vi "Inline - Update Status Channels.vi"(7 "Status Channel":T1, 8 "Error Code":i32, 9 "Time (us)":u32, 11 "RTStateVariables":T2 {"Inline Status Channels Refs" format="%.0x"; "Rx Config"."Labels Settings"."Label Timestamp Channel Data Reference" format="%.0x"; "Rx Config"."Labels Settings"."Label Disable/Trigger Channel Reference" format="%.0x"; "Rx Config"."Labels Settings"."Label" format="%.0o"}) -> ()   [LabVIEW 2020, in "Ballard Arinc-429 Engine.lvlib"]
doc: "This VI updates some Inline Status Channels."
uses:
  Ballard Arinc-429 Engine.lvlib
  RT Controls/RTStateVariables.ctl
  <vilib>/NI/NIVS Inline Async API/_VS Inline Async API/VS Inline Async API/VS Inline Async API.lvclass
  RT Controls/Card Parameters.ctl
  Shared/Controls and Global/Initialization Method.ctl
  Shared/Controls and Global/RT HW Channel.ctl
  Shared/Controls and Global/RT Label Settings.ctl
  Shared/Controls and Global/Label.ctl
  Shared/Controls and Global/transferPeriod.ctl
  Shared/Controls and Global/RT Word Settings.ctl
  Shared/Controls and Global/RT Param Setting.ctl
  Shared/Controls and Global/Start Bit.ctl
  Shared/Controls and Global/Number of Bits.ctl
  <vilib>/NI VeriStand/Custom Device API/Block Data Reference.ctl
  <vilib>/NI VeriStand/Custom Device API/Data Reference.ctl
  <vilib>/NI VeriStand/Custom Device API/Custom Device Item Ref.ctl
  Shared/Controls and Global/TransferType.ctl
  RT Controls/Inline_Status_Channels.ctl
  <vilib>/NI VeriStand/Custom Device API/Global Data Refs.vi
  <vilib>/NI VeriStand/Custom Device API/Custom Device API.lvlib
  Shared/Ballard Arinc-429 Shared.lvlib
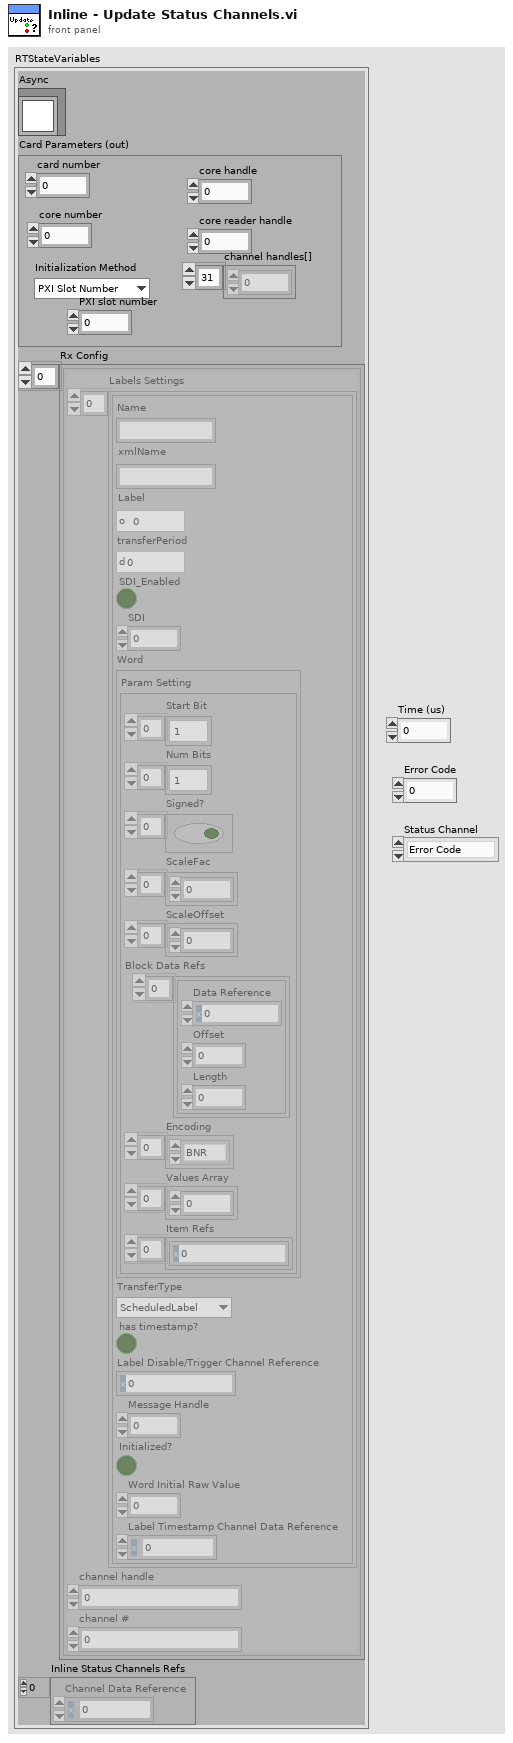
[diagram p1: front panel]
types:
  T1 = typedef "Ballard Arinc-429 Engine.lvlib/Inline_Status_Channels.ctl" = enum16{"Error Code", "Inline Read Time (us)", "Inline Write Time (us)", "Receiving Error - Error Counter", "Gap Error - Error Counter", "Parity Error - Error Counter", "Long Word Error - Error Counter", "Bit Timing Error - Error Counter"}
  T2 = typedef "Ballard Arinc-429 Engine.lvlib/RTStateVariables.ctl" = cluster{"Async":refnum<class "VS Inline Async API.lvclass">, "Card Parameters (out)":T3, "Rx Config":T5[], "Inline Status Channels Refs":T14[]}
  T3 = typedef "Ballard Arinc-429 Engine.lvlib/Card Parameters.ctl" = cluster{"card number":i32, "core number":i32, "core handle":u64, "core reader handle":u64, "channel handles[]":u64[], "Initialization Method":T4, "PXI slot number":i32}
  T4 = typedef "Ballard Arinc-429 Shared.lvlib/Initialization Method.ctl" = enum16{"PXI Slot Number", "Card Number"}
  T5 = typedef "Ballard Arinc-429 Shared.lvlib/RT HW Channel.ctl" = cluster{"Labels Settings":T6[], "channel handle":u64, "channel #":u16}
  T6 = typedef "Ballard Arinc-429 Shared.lvlib/RT Label Settings.ctl" = cluster{"Name":string, "xmlName":string, "Label":T7, "transferPeriod":T8, "SDI_Enabled":bool, "SDI":u8, "Word":T9, "TransferType":T16, "has timestamp?":bool, "Label Disable/Trigger Channel Reference":T15, "Message Handle":u64, "Initialized?":bool, "Word Initial Raw Value":u32, "Label Timestamp Channel Data Reference":T14}
  T7 = typedef "Ballard Arinc-429 Shared.lvlib/Label.ctl" = u8
  T8 = typedef "Ballard Arinc-429 Shared.lvlib/transferPeriod.ctl" = u32
  T9 = typedef "Ballard Arinc-429 Shared.lvlib/RT Word Settings.ctl" = cluster{"Param Setting":T10}
  T10 = typedef "Ballard Arinc-429 Shared.lvlib/RT Param Setting.ctl" = cluster{"Start Bit":T11[], "Num Bits":T12[], "Signed?":bool[], "ScaleFac":dbl[], "ScaleOffset":dbl[], "Block Data Refs":T13[], "Encoding":enum16{"BNR", "BCD", "Discrete"}[], "Values Array":dbl[], "Item Refs":T15[]}
  T11 = typedef "Ballard Arinc-429 Shared.lvlib/Start Bit.ctl" = i32
  T12 = typedef "Ballard Arinc-429 Shared.lvlib/Number of Bits.ctl" = i32
  T13 = typedef "Custom Device API.lvlib/Block Data Reference.ctl" = cluster{"Data Reference":T14, "Offset":u64, "Length":u64}
  T14 = typedef "Custom Device API.lvlib/Data Reference.ctl" = i32
  T15 = typedef "Custom Device API.lvlib/Custom Device Item Ref.ctl" = u64
  T16 = typedef "Ballard Arinc-429 Shared.lvlib/TransferType.ctl" = enum16{"ScheduledLabel", "Acyclic", "Block", "Strobe"}
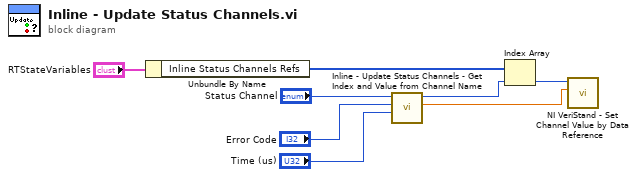
[diagram p0: block diagram]
diagram:
  n1 = Unbundle By Name("RTStateVariables") -> ("Inline Status Channels Refs"=w7:T14[])
  n2 = call "Inline - Update Status Channels - Get Index and Value from Channel Name.vi"("Time (us)/Error Counter Value"="Time (us)", "Error Code"="Error Code", "Status Channel"="Status Channel") -> ("Value"=w2:dbl, "index"=w6:i32)  [unwired: 7 in]
  n3 = Index Array(array=w7, index=w6) -> (element=w5:T14)
  n4 = call <vilib>:"NI VeriStand - Set Channel Value by Data Reference.vi"("Value"=w2, "Data Reference in"=w5) -> ()  [unwired: 9 in, 1 out]
